vi "Math-Mask Runs.vi"(1 "Min Run Length":i32=2, 2 "Array":bool[](array[boolean])) -> (0 "Runs Mask":bool[](array[boolean]))   [LabVIEW 2020]
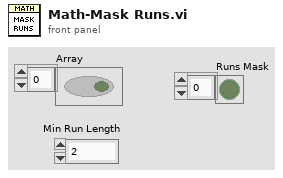
[diagram p1: front panel]
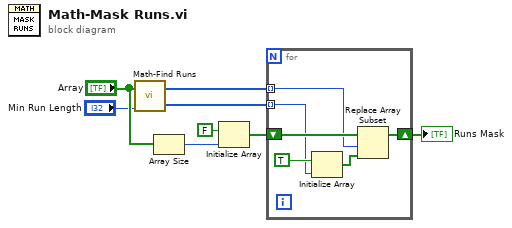
[diagram p0: block diagram]
diagram:
  n1 = call "Math-Find Runs.vi"("Min Run Length"="Min Run Length", "Array"="Array") -> ("Length"=w4:i32[], "Start"=w3:i32[])
  n2 = Array Size(array="Array") -> (size(s)=w6:i32)
  n3 = Initialize Array(FALSE, w6) -> (w8:bool[])
  n4 = for {
    tunnel: w3 -> [w12] mode=indexing
    tunnel: w4 -> [w9] mode=indexing
    shift-right: [w13] -> w1
    shift-left: w8 -> [w14]
    n5 = Initialize Array(TRUE, w9) -> (w10:bool[])
    n6 = Replace Array Subset(array=w14, new element=w10, index=w12) -> (w13:bool[])
  }
  "Runs Mask" <- w1
